vi "RSZVB Configure External Power Meter.vi"(5 "Power Meter Type":string, 6 "Interface Address":string, 7 "Interface Type":string, 8 "error in (no error)":errorcluster {"code" format="%.0x"}, 9 "Power Meter Name":string, 10 "Power Meter Number (1)":i32=1, 11 "VISA session":refnum<visa-resource-name>) -> (0 "error out":errorcluster {"code" format="%.0x"}, 3 "dup VISA session":refnum<visa-resource-name>)   [LabVIEW 2011]
doc: "This VI configures an external power meter and adds it to the list of available power meters.\n\nRemote-control command(s):\nSYSTem:COMMunicate:RDEVice:PMETer<pmeter_no>:DEFine\n'<pmeter_name>', '<driver>', '<interface>', '<address>'"
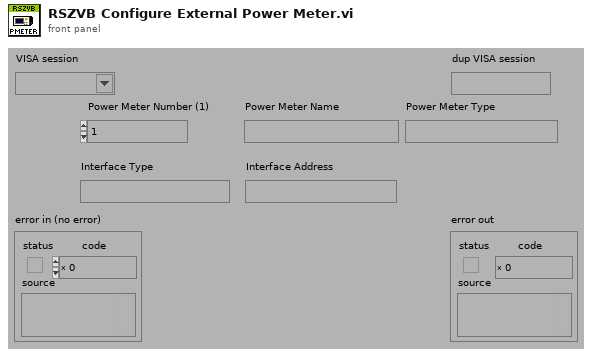
[diagram p1: front panel]
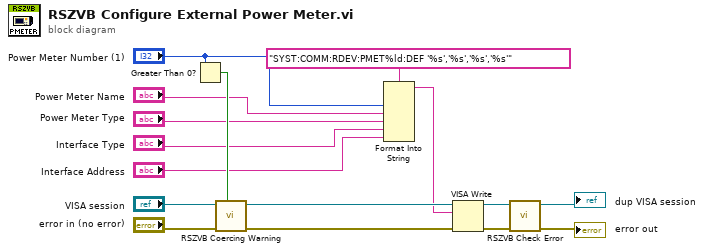
[diagram p0: block diagram]
diagram:
  n1 = Greater Than 0?(x="Power Meter Number (1)") -> (x > 0?=w12:bool)
  n2 = call "RSZVB Coercing Warning.vi"("In Range?"=w12, "error in (no error)"="error in (no error)", "VISA session"="VISA session") -> ("error out"=w15:errorcluster, "dup VISA session"=w16:refnum<visa-resource-name>)  [unwired: 7 in]
  n3 = Format Into String(format string="SYST:COMM:RDEV:PMET%ld:DEF '%s','%s','%s','%s'", "Power Meter Number (1)", "Power Meter Name", "Power Meter Type", "Interface Type", "Interface Address") -> (resulting string=w10:string)  [unwired: 2 in, 1 out]
  n4 = VISA Write(VISA resource name=w16, write buffer=w10, error in (no error)=w15) -> (VISA resource name out=w13:refnum<visa-resource-name>, error out=w14:errorcluster)  [unwired: 1 out]
  n5 = call "RSZVB Check Error.vi"("error in (no error)"=w14, "VISA session"=w13) -> ("error out"=→"error out":errorcluster, "dup VISA session"=→"dup VISA session":refnum<visa-resource-name>)  [unwired: 8 in]
